vi "dfd_Judge Special String.vi"(11 "string":string) -> (2 "separator":bool, 3 "space ?":bool)   [LabVIEW 2017, in "NI_DigFilter_Process.lvlib"]
uses:
  <vilib>/addons/Digital Filter Design/NI_DigFilter_Process.lvlib
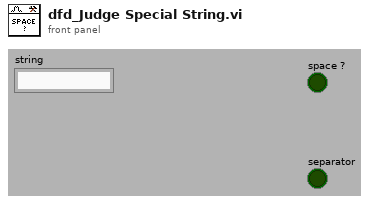
[diagram p1: front panel]
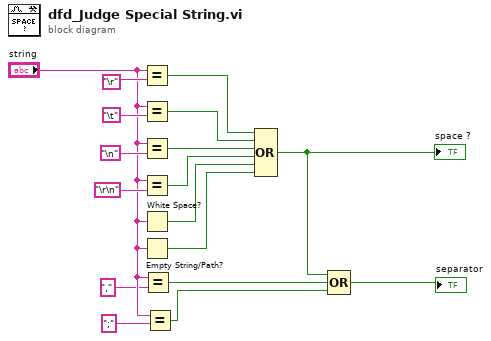
[diagram p0: block diagram]
diagram:
  n1 = Equal?(x="string", y="\r") -> (x = y?=w7:bool)
  n2 = Equal?(x="string", y="\t") -> (x = y?=w5:bool)
  n3 = Equal?(x="string", y="\n") -> (x = y?=w4:bool)
  n4 = Equal?(x="string", y="\r\n") -> (x = y?=w3:bool)
  n5 = White Space?(1:"string") -> (0:w2:bool)
  n6 = Empty String/Path?(string/path="string") -> (empty?=w1:bool)
  n7 = Equal?(x="string", y=",") -> (x = y?=w10:bool)
  n8 = Equal?(x="string", y=";") -> (x = y?=w9:bool)
  n9 = Compound Arithmetic op=OR(w7, w5, w4, w3, w2, w1) -> (w6:bool)
  "space ?" <- w6
  n10 = Compound Arithmetic op=OR(w6, w10, w9) -> (→"separator":bool)
